vi "Performance Test.vi"() -> ()   [LabVIEW 2021]
uses:
  ChannelCommon/typedef/Benchmark Stats.ctl
  ChannelCommon/typedef/Datatype Waveform.ctl
  CIFChannels/Typedef/Direction.ctl
  ChannelCommon/typedef/FIFO Config.ctl
  CIF_DAQ_DVR_Multi.lvclass
  D:/dev/Packages/Channel_Manager/src/CIFChannels/CIFChannels.lvclass
  ChannelCommon/typedef/New FIFO Instance Configuration.ctl
  <vilib>/Platform/TimedLoop/XDataNode/timing_clust.ctl
  <vilib>/Platform/TimedLoop/XDataNode/nitl_modes.ctl
  <vilib>/Platform/TimedLoop/XDataNode/wakeup.ctl
  ChannelCommon/typedef/TimeStamps.ctl
  CIFChannels/CIFChannels.lvclass/CIFChannels.ctl
  <vilib>/CIF Foundation/CIF Utilities/Statistics/I64/Stats_I64_CIF_U.lvclass/Stats_I64_CIF_U.ctl
  <vilib>/CIF Foundation/CIF Utilities/DataTypes/Flatten U64.vi
  <vilib>/CIF Foundation/CIF Utilities/Statistics/I64/Get Stats.vi
  <vilib>/Platform/TimedLoop/XDataNode/XDataNode.xnode
  <vilib>/Platform/TimedLoop/XDataNode/XDNodeRunTimeDep.lvlib
  CIFChannels/CIFChannels.lvclass
  ChannelCommon/ChannelCommon.lvlib
panel:
  out "Timeout RW Inline":bool
  out "Write (us) 3":T1
  out "Flatten (us) 3":T1
  out "Data Out":T2[](array[typedef])=[{"measurement"=array[200001 elements], "dT"=43.0, "Timestamp"=2, "Read Lock"=FALSE}, {"measurement"=array[200001 elements], "dT"=34.0, "Timestamp"=1, "Read Lock"=FALSE}]
  out "Read (us) 3":T1
  out "Unflatten (us) 3":T1
  out "pass":bool
  out "error out":errorcluster
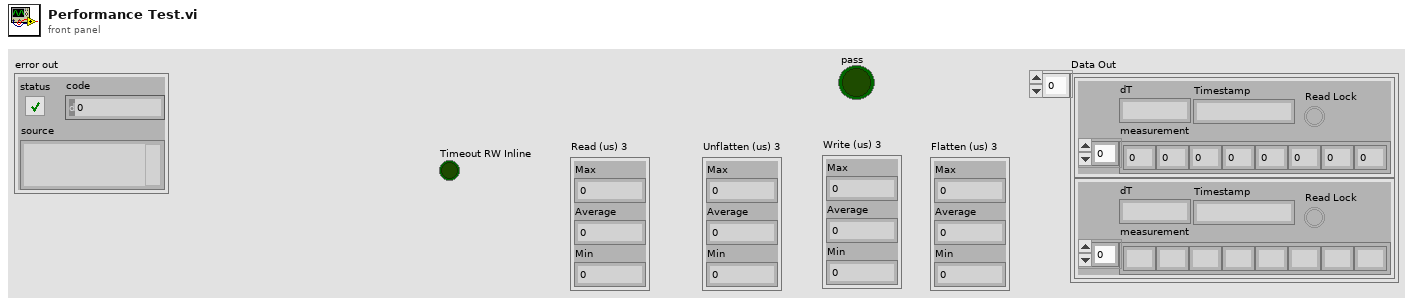
[diagram p1: front panel]
types:
  T1 = typedef "ChannelCommon.lvlib/Benchmark Stats.ctl" = cluster{"Max":i64, "Average":dbl, "Min":i64}
  T2 = typedef "ChannelCommon.lvlib/Datatype Waveform.ctl" = cluster{"measurement":dbl[], "dT":dbl, "Timestamp":i64, "Read Lock":bool}
  T3 = typedef "ChannelCommon.lvlib/FIFO Config.ctl" = cluster{"Max Bytes/Msg":u64, "Max Msg/FIFO":u64, "Flags":u64}
  T4 = typedef "CIFChannels.lvclass/Direction.ctl" = enum16{"Publisher", "Subscriber"}
  T5 = typedef "ChannelCommon.lvlib/New FIFO Instance Configuration.ctl" = cluster{"Primary":bool, "Backpressure":bool, "Message/FIFO Override":u32}
  T6 = typedef "ChannelCommon.lvlib/TimeStamps.ctl" = cluster{"ClockID":u8, "T0":i64, "T_Out":i64}
  T7 = typedef "XDNodeRunTimeDep.lvlib/timing_clust.ctl" = cluster{"Expected End [f-1]":u64, "Actual End [f-1]":u64, "Finished Late? [f-1]":bool, "Expected End [i-1]":u64, "Actual End [i-1]":u64, "Finished Late? [i-1]":bool, "Expected Start [i]":u64, "Actual Start [i]":u64, "Expected Start [f]":u64, "Actual Start [f]":u64, "Source Name":string, "Structure Name":string, "Period":i64, "Deadline":i64, "Offset":i64, "Start":i64, "Priority":i32, "Timeout":i32, "Mode":T8, "Wakeup Reason":T9, "Error":errorcluster, "Source Type":string, "Secondary Source Type":string, "Global End Time":u64, "Global Start Time":u64, "Frame Duration":u64, "Iteration Duration":u64, "Assigned CPU":i32, "I/O Scan Engine Mode":u32}
  T8 = typedef "XDNodeRunTimeDep.lvlib/nitl_modes.ctl" = enum32{"No Change", "Process missed periods, maintain original phase", "Discard missed periods, maintain original phase", "Process missed periods, ignore original phase", "Discard missed periods, ignore original phase"}
  T9 = typedef "XDNodeRunTimeDep.lvlib/wakeup.ctl" = enum32{"Normal", "Aborted", "Asynchronous wakeup", "Timing source error", "Timed loop error", "Timeout"}
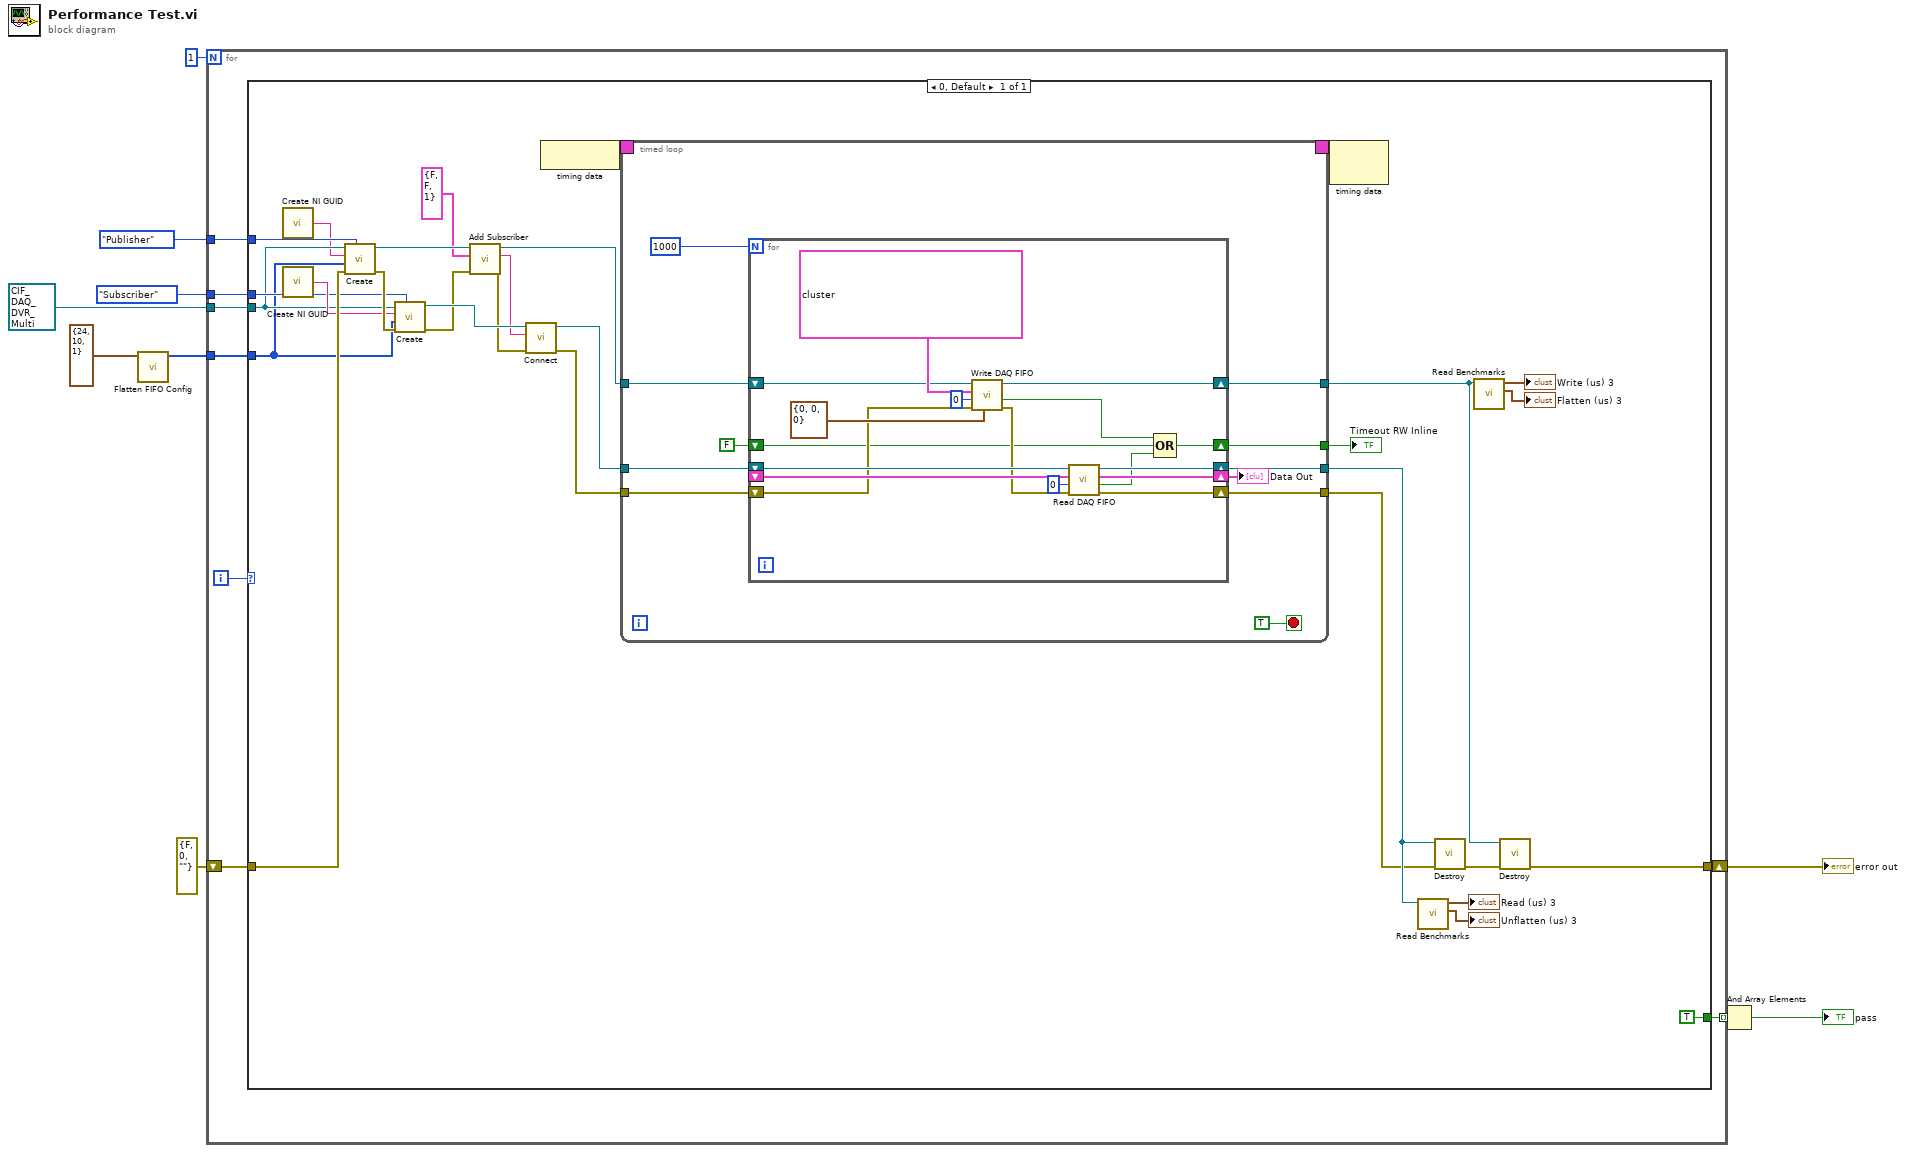
[diagram p0: block diagram]
diagram:
  n1 = call "Flatten FIFO Config.vi"("FIFO Config in"=T3 {"Max Bytes/Msg"=24, "Max Msg/FIFO"=10, "Flags"=1}) -> ("Flattened FIFO Config"=w2:u8[])  [unwired: 10 in]
  n2 = for {
    N: 1 -> [_]
    tunnel: [w18] -> w8 mode=indexing
    shift-right: [w17] -> w10
    shift-left: errorcluster {"status"=FALSE, "code"=0, "source"=""} ("error out") -> [w15]
    tunnel: Direction."Publisher" ("Direction") -> [w14]
    tunnel: Direction."Subscriber" ("Direction") -> [w13]
    tunnel: refnum<class "CIF_DAQ_DVR_Multi.lvclass"> refnum ("CIF_DAQ_DVR_Multi.lvclass") -> [w12]
    tunnel: w2 -> [w11]
    i -> [w16]
    n3 = case shown="0, Default" w16 {
      tunnel: [TRUE] -> w18
      tunnel: [w38] -> w17
      tunnel: w15 -> [w47]
      tunnel: w14 -> [w45]
      tunnel: w13 -> [w44]
      tunnel: w12 -> [w43]
      tunnel: w11 -> [w40]
      frame 0, Default {
        n4 = call <vilib>:"Create NI GUID.vi"() -> ("NI GUID"=w41:string)
        n5 = call <vilib>:"Create NI GUID.vi"() -> ("NI GUID"=w46:string)
        n6 = call-dynamic "Create.vi"("Direction"=w45, "error in (no error)"=w47, "Custom Config Data"=w40, "Name"=w41, "CIF_DAQ_DVR_Multi in"=w43) -> ("error out"=w48:errorcluster, "CIF_DAQ_DVR_Multi out"=w24:refnum<class "CIF_DAQ_DVR_Multi.lvclass">)  [unwired: 5 in]
        n7 = call-dynamic "Create.vi"("Direction"=w44, "error in (no error)"=w48, "Custom Config Data"=w40, "Name"=w46, "CIF_DAQ_DVR_Multi in"=w43) -> ("error out"=w20:errorcluster, "CIF_DAQ_DVR_Multi out"=w42:refnum<class "CIF_DAQ_DVR_Multi.lvclass">)  [unwired: 5 in]
        n8 = call "Add Subscriber.vi"("error in (no error)"=w20, "New FIFO Instance Config"=T5 {"Primary"=FALSE, "Backpressure"=FALSE, "Message/FIFO Override"=1}, "CIF_DAQ_DVR_Multi in"=w24) -> ("error out"=w19:errorcluster, "New Publisher"=w21:string, "CIF_DAQ_DVR_Multi out"=w23:refnum<class "CIF_DAQ_DVR_Multi.lvclass">)  [unwired: 6 in]
        n9 = call-dynamic "Connect.vi"("error in (no error)"=w19, "Connection Name"=w21, "CIFTag in"=w42) -> ("error out"=w32:errorcluster, "CIFTag out"=w33:refnum<class "CIF_DAQ_DVR_Multi.lvclass">)  [unwired: 7 in]
        n10 = node-c288() -> (w35:T7)
        n11 = timed-loop {
          timing: w35 -> [_]
          timing-out: [_] -> w34
          tunnel: w33 -> [w59]
          tunnel: w32 -> [w58]
          tunnel: [w56] -> w31
          tunnel: [w55] -> w30
          tunnel: [w50] -> w25
          tunnel: w23 -> [w53]
          tunnel: [w52] -> w27
          stop <- TRUE stop-if-true
          n12 = for {
            N: 1000 -> [_]
            shift-right: [w72] -> w56
            shift-left: w59 -> [w76]
            shift-right: [w75] -> w55
            shift-left: w58 -> [w69]
            shift-right: [w74] -> w49
            shift-left: _ -> [w73]
            shift-right: [w66] -> w52
            shift-left: w53 -> [w67]
            shift-right: [w61] -> w50
            shift-left: FALSE -> [w62]
            n13 = call-dynamic "Write DAQ FIFO.vi"("FIFO Timestamps"=T6 {"ClockID"=0, "T0"=0, "T_Out"=0}, "error in (no error)"=w69, "Timeout (ms)"=0, "Data In"=T2[] [{"measurement"=array[200001 elements], "dT"=43.0, "Timestamp"=2, "Read Lock"=FALSE}, {"measurement"=array[200001 elements], "dT"=34.0, "Timestamp"=1, "Read Lock"=FALSE}] ("DAQ In"), "CIF_DAQ_DVR_Multi in"=w67) -> ("error out"=w68:errorcluster, "timed out?"=w60:bool, "CIF_DAQ_DVR_Multi out"=w66:refnum<class "CIF_DAQ_DVR_Multi.lvclass">)  [unwired: 3 in, 1 out]
            n14 = call-dynamic "Read DAQ FIFO.vi"("error in (no error)"=w68, "Timeout (ms)"=0, "Data In"=w73, "CIF_NIChn_FIFO_DAQ in"=w76) -> ("error out"=w75:errorcluster, "timed out?"=w63:bool, "Data Out"=w74:T2[], "CIF_NIChn_FIFO_DAQ out"=w72:refnum<class "CIF_DAQ_DVR_Multi.lvclass">)  [unwired: 3 in, 1 out]
            n15 = Compound Arithmetic op=OR(w60, w62, w63) -> (w61:bool)
          }
          "Data Out" <- w49
        }
        "Timeout RW Inline" <- w25
        n16 = node-c288(w34) -> ()  [unwired: 1 out]
        n17 = call "Read Benchmarks.vi"("CIFChannels in"=w31) -> ("Flatten (us)"=→"Unflatten (us) 3":T1, "Channel R/W (us)"=→"Read (us) 3":T1)  [unwired: 9 in]
        n18 = call-dynamic "Destroy.vi"("error in (no error)"=w30, "CIF_DAQ_DVR_Multi in"=w31) -> ("error out"=w39:errorcluster)  [unwired: 8 in, 1 out]
        n19 = call "Read Benchmarks.vi"("CIFChannels in"=w27) -> ("Flatten (us)"=→"Flatten (us) 3":T1, "Channel R/W (us)"=→"Write (us) 3":T1)  [unwired: 9 in]
        n20 = call-dynamic "Destroy.vi"("error in (no error)"=w39, "CIF_DAQ_DVR_Multi in"=w27) -> ("error out"=w38:errorcluster)  [unwired: 8 in, 1 out]
      }
    }
  }
  "error out" <- w10
  n21 = And Array Elements(Boolean array=w8) -> (logical AND=→"pass":bool)
